vi "TDMS Read Property Value (String).vi"(2 "Property Name":string, 3 "Property Names":string[](array[string]), 4 "Property Values":variant[](array[variant])) -> (0 "Found?":bool, 1 "Property Value":string)   [LabVIEW 2011]
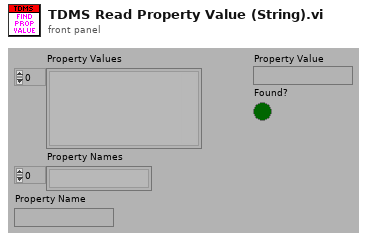
[diagram p1: front panel]
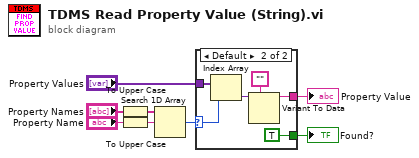
[diagram p0: block diagram]
diagram:
  n1 = To Upper Case(1:"Property Names") -> (0:w3:string[])
  n2 = To Upper Case(1:"Property Name") -> (0:w2:string)
  n3 = Search 1D Array(1D array=w3, element=w2) -> (index of element=w7:i32)  [unwired: 1 out]
  n4 = case shown="Default" w7 {
    selector: w7 -> [_ w13]
    tunnel: "Property Values" -> [_ w14]
    tunnel: [_ w10] -> w6
    tunnel: [_ TRUE ("Found?")] -> w1
    frame -1 {
    }
    frame Default {
      n5 = Index Array(array=w14, index=w13) -> (element=w12:variant)
      n6 = Variant To Data(type="", Variant=w12) -> (data=w10:string)  [unwired: 1 in, 1 out]
    }
  }
  "Property Value" <- w6
  "Found?" <- w1
